vi "ZedBoardControls.vi"(4 "Register Map\nDefaults":refnum<vi>, 6 "Register Map\nRead Ref":refnum<vi>, 7 "NewRegMapReady":refnum<vi>, 8 "Last Command\nSent Ref":refnum<vi>, 9 "Stop Loop \nRef":refnum<vi>, 10 "error out":errorcluster, 11 "queue out":refnum<queue>) -> ()   [LabVIEW 2012]
panel:
  in  "Power Pulse\nReject Config":u16
  in  "Power Mon \nAcc Mode":string(combo)
  in  "Power Mon Test Mode":string(combo)
  in  "Power Mon Chan Enable":bool[](array[boolean])
  out "word9":string
  in  "Send Word A":bool
  in  "SoftDEMUX \nSelector Enable":bool
  in  "Sync Select 3B":string(combo)
  in  "Sync Select 2B":string(combo)
  in  "Sync Select 1B":string(combo)
  in  "Sync Select 0B":string(combo)
  in  "Sync Select 7":string(combo)
  in  "Sync Select 6":string(combo)
  in  "Sync Select 5":string(combo)
  in  "Sync Select 4":string(combo)
  in  "Sync Select 3A":string(combo)
  in  "Sync Select 2A":string(combo)
  in  "Sync Select 1A":string(combo)
  in  "Sync Select 0A":string(combo)
  in  "Sync Test\nMode Config":u32
  in  "Pulse Period\n(clock cycles -1)":u32
  in  "Channel DEMUX \nSelector":bool
  in  "Channel \nHold Order":bool
  in  "Channel \nTransfer Order":bool
  in  "Throttle Mode":string(combo)
  in  "Sync Test Mode Select":string(combo)
  in  "Data Input Test Mode":string(combo)
  out "Last Command Sent":string
  in  "Reset Channel Enable":bool
  in  "Send Command, manual entry":string
  in  "Send":bool
  in  "Read Register":bool
  in  "Reset Register Map to Defaults":bool
  in  "Sync Enable":bool[](array[boolean])
  in  "Channel Enable":bool[](array[boolean])
  in  "Reset Profile Accumulator":bool[](array[boolean])
  in  "Counts Per Bin":u16
  in  "User Reset":bool
  in  "Number of Bins":u16
  in  "Profiles Per Histogram":u16
  in  "Time Reset":bool
  in  "Relative Time Step":u32
  in  "Demux Channel Enable":bool[](array[boolean])
  out "word0":string
  out "word1":string
  out "word2":string
  out "word3":string
  out "word4":string
  out "word5":string
  out "word6":string
  out "word7":string
  out "word8":string
  in  "DIN Polarity":bool[](array[boolean])
  in  "DIN Demux Polarity":bool[](array[boolean])
  in  "Sync Input Polarity":bool[](array[boolean])
  in  "PIN0 Pulse Durration Ave 2^N":u16
  out "wordA":string
  in  "PIN1 Pulse Durration Ave 2^N":u16
  in  "PIN2 Pulse Durration Ave 2^N":u16
  in  "PIN3 Pulse Durration Ave 2^N":u16
  in  "PIN4 Pulse Durration Ave 2^N":u16
  in  "PIN5 Pulse Durration Ave 2^N":u16
  in  "Send Word 0":bool
  in  "Send Word 1":bool
  in  "Send Word 2":bool
  in  "Send Word 3":bool
  in  "Send Word 4":bool
  in  "Send Word 5":bool
  in  "Send Word 6":bool
  in  "Send Word 7":bool
  in  "Send Word 8":bool
  in  "Send Word 9":bool
  # "word0"
  # "word1"
  # "word2"
  # "word3"
  # "word4"
  # "valid range (2-4096)"
  # "valid range (2-4096)"
  # "valid range (1-32,768)"
  # "word5"
  # "word6"
  # "valid range (0-256)"
  # "valid range (0-64)"
  # "word7"
  # "word8"
  # "word9"
  # "valid range (0-33,554,432)"
  # "valid range (0-256)"
  # "wordA"
  # "N=valid range (0-15)"
  # "N=valid range (0-15)"
  # "N=valid range (0-15)"
  # "N=valid range (0-15)"
  # "N=valid range (0-15)"
  # "N=valid range (0-15)"
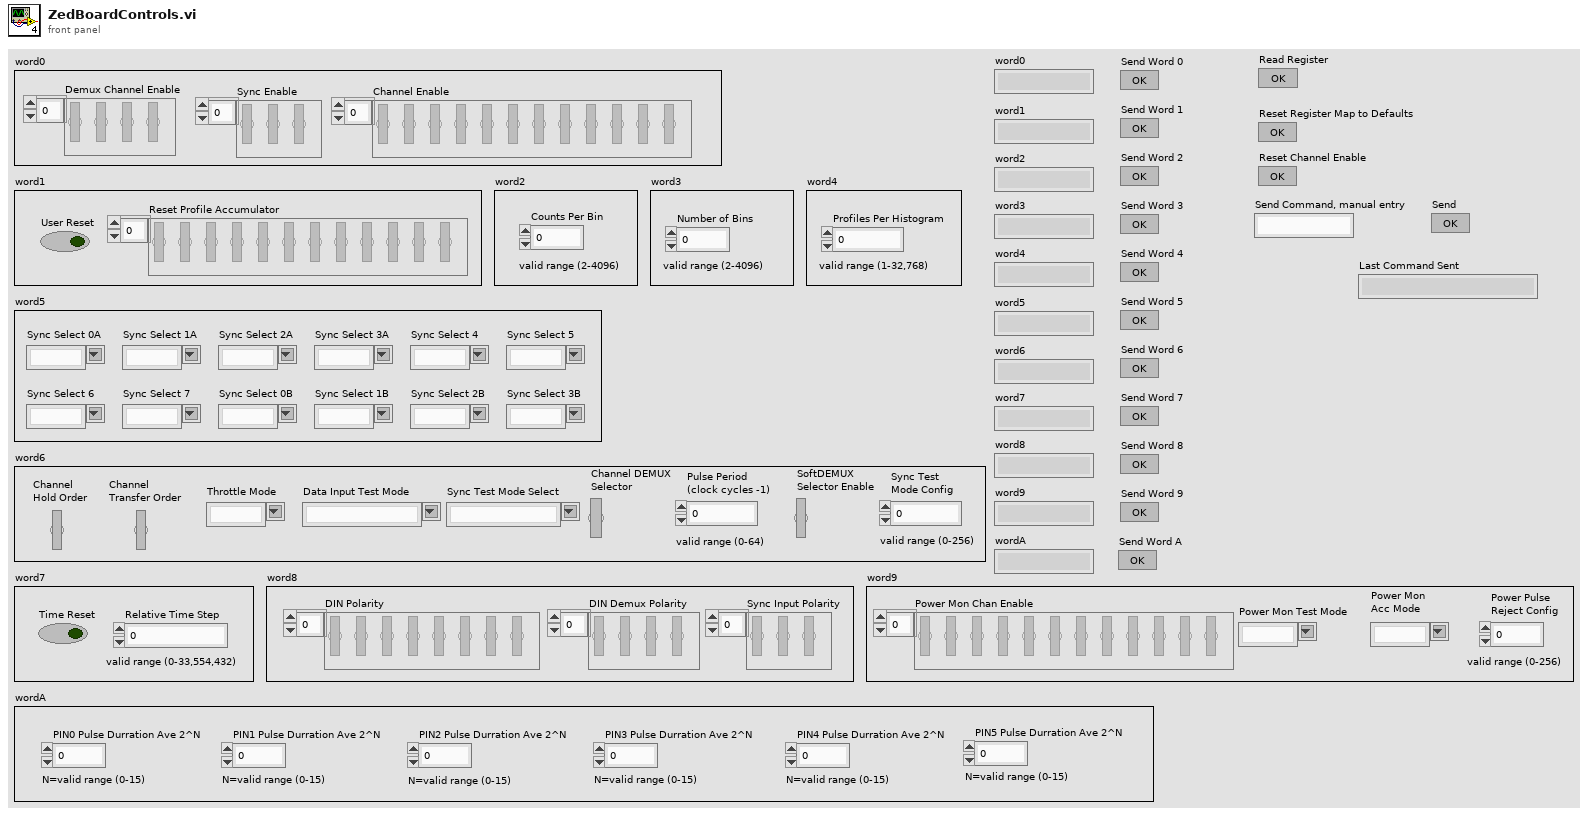
[diagram p1: front panel]
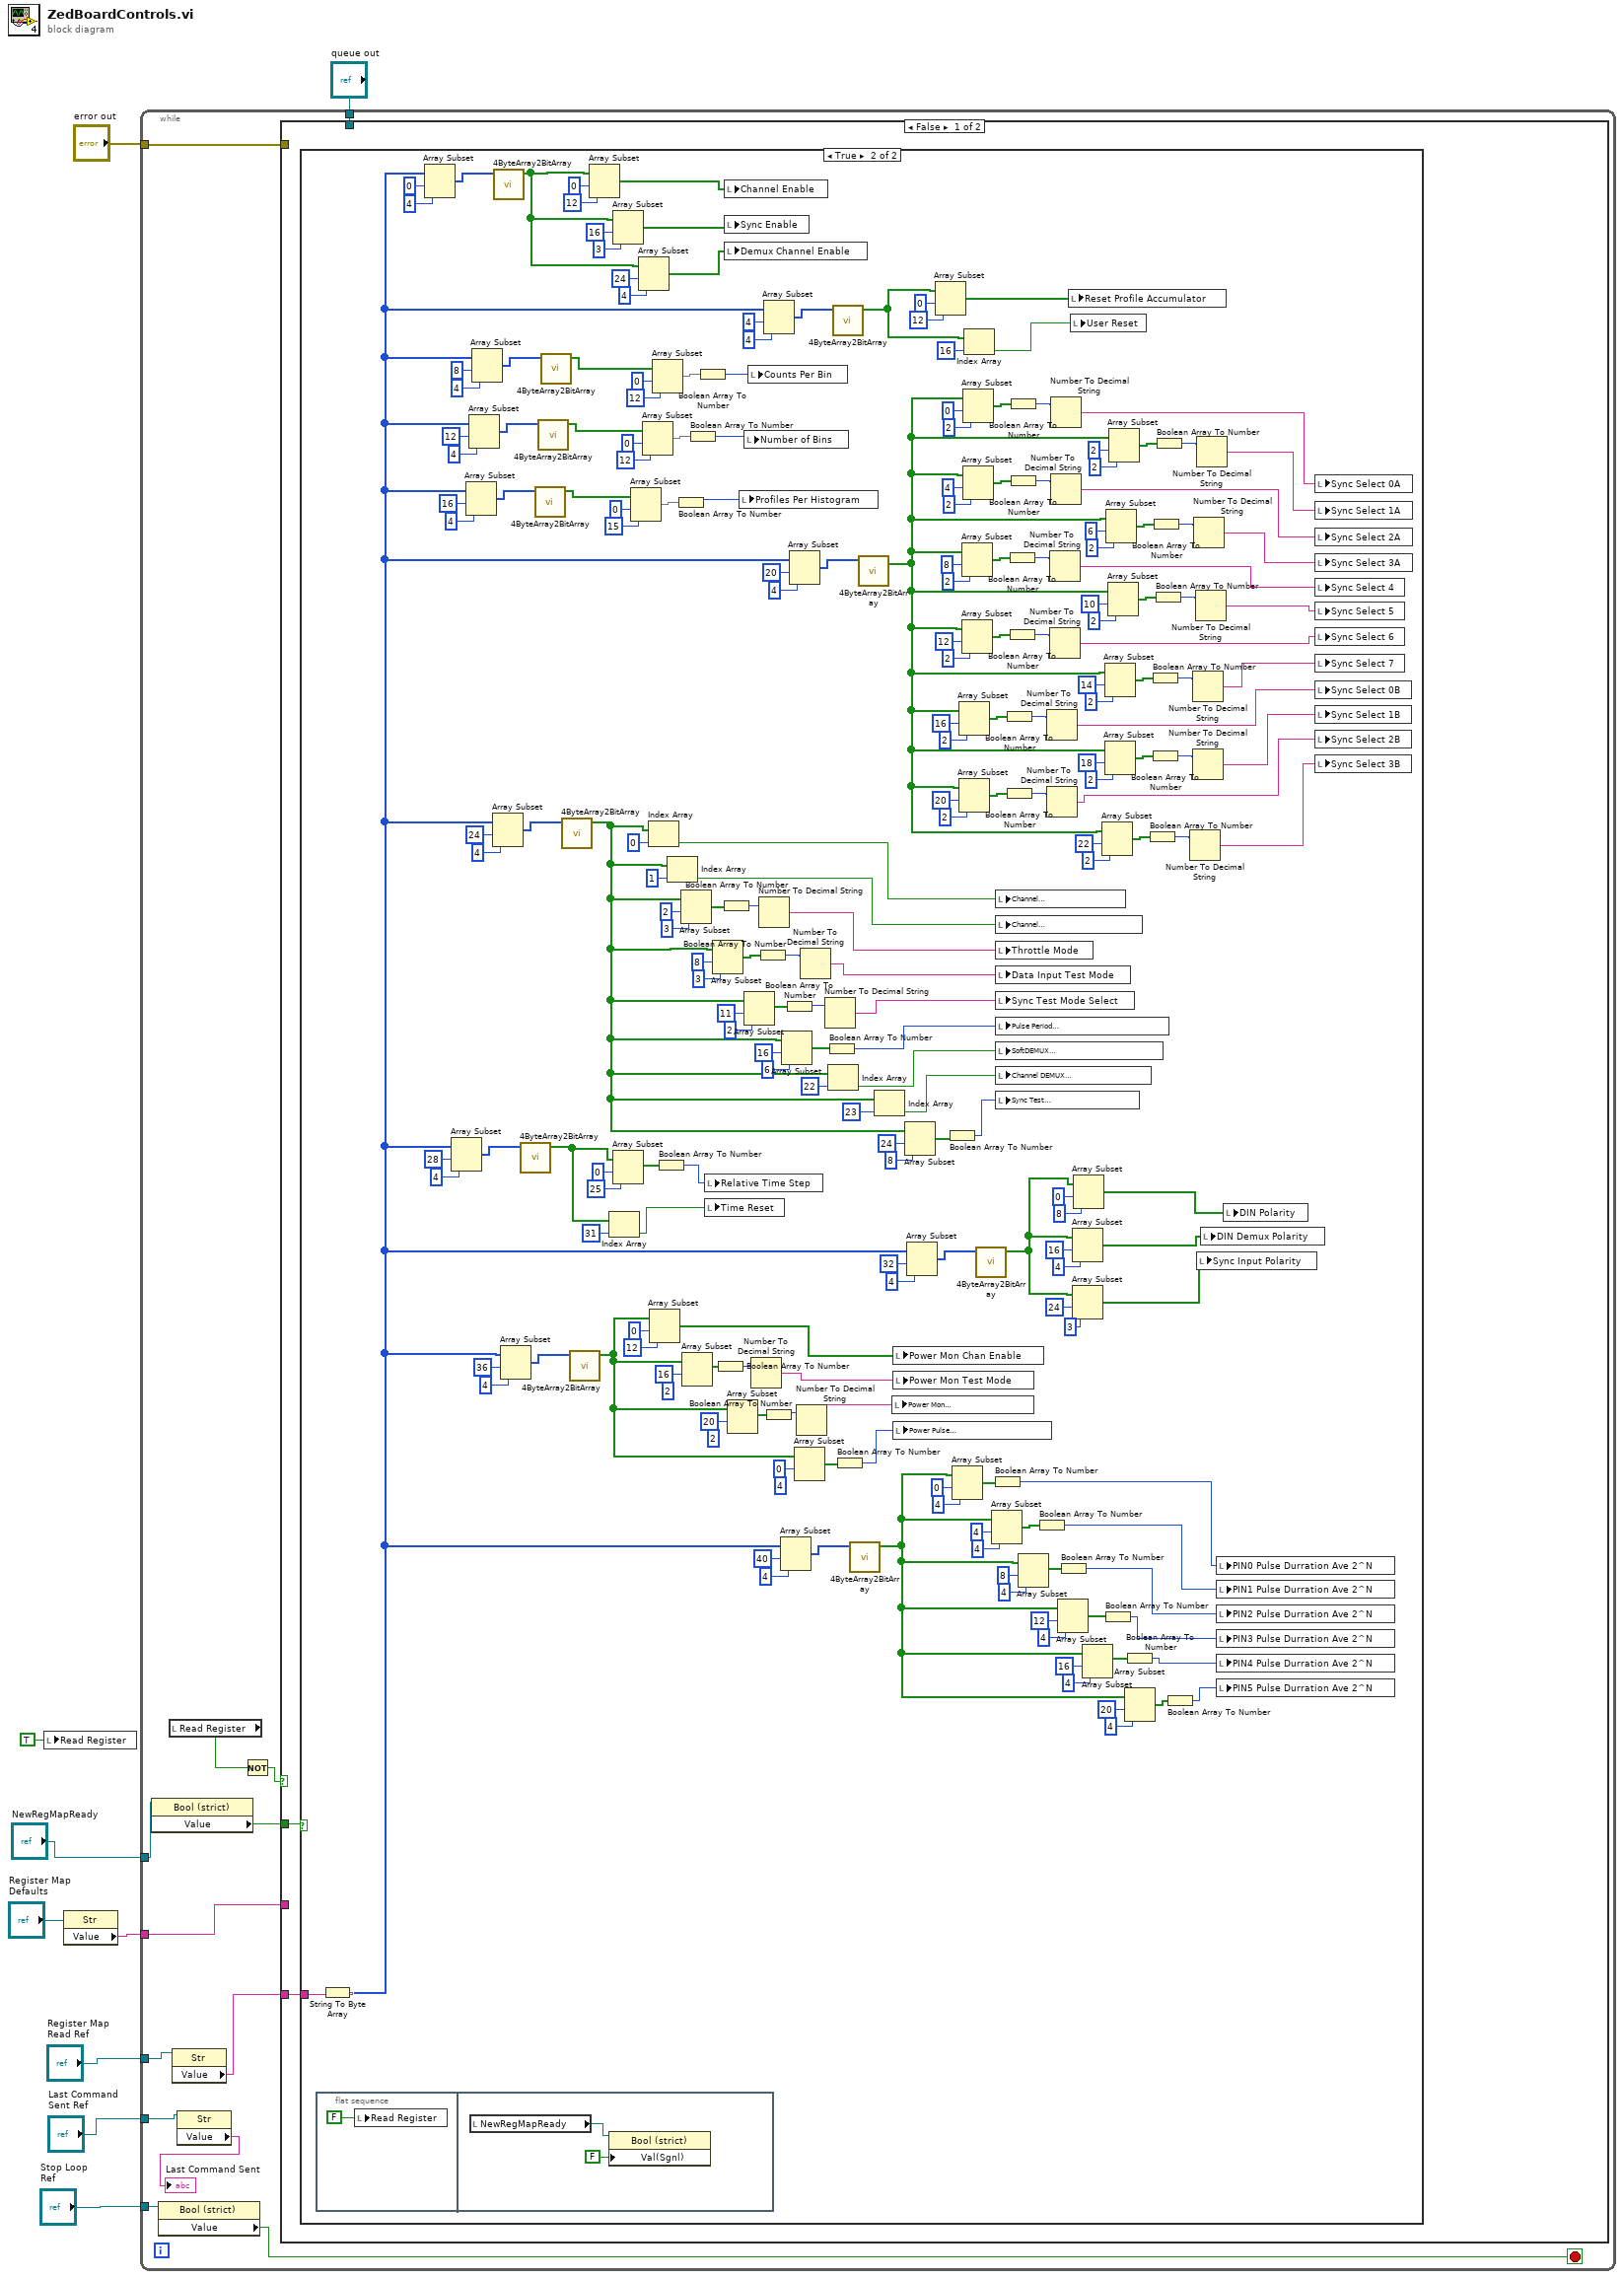
[diagram p0: block diagram]
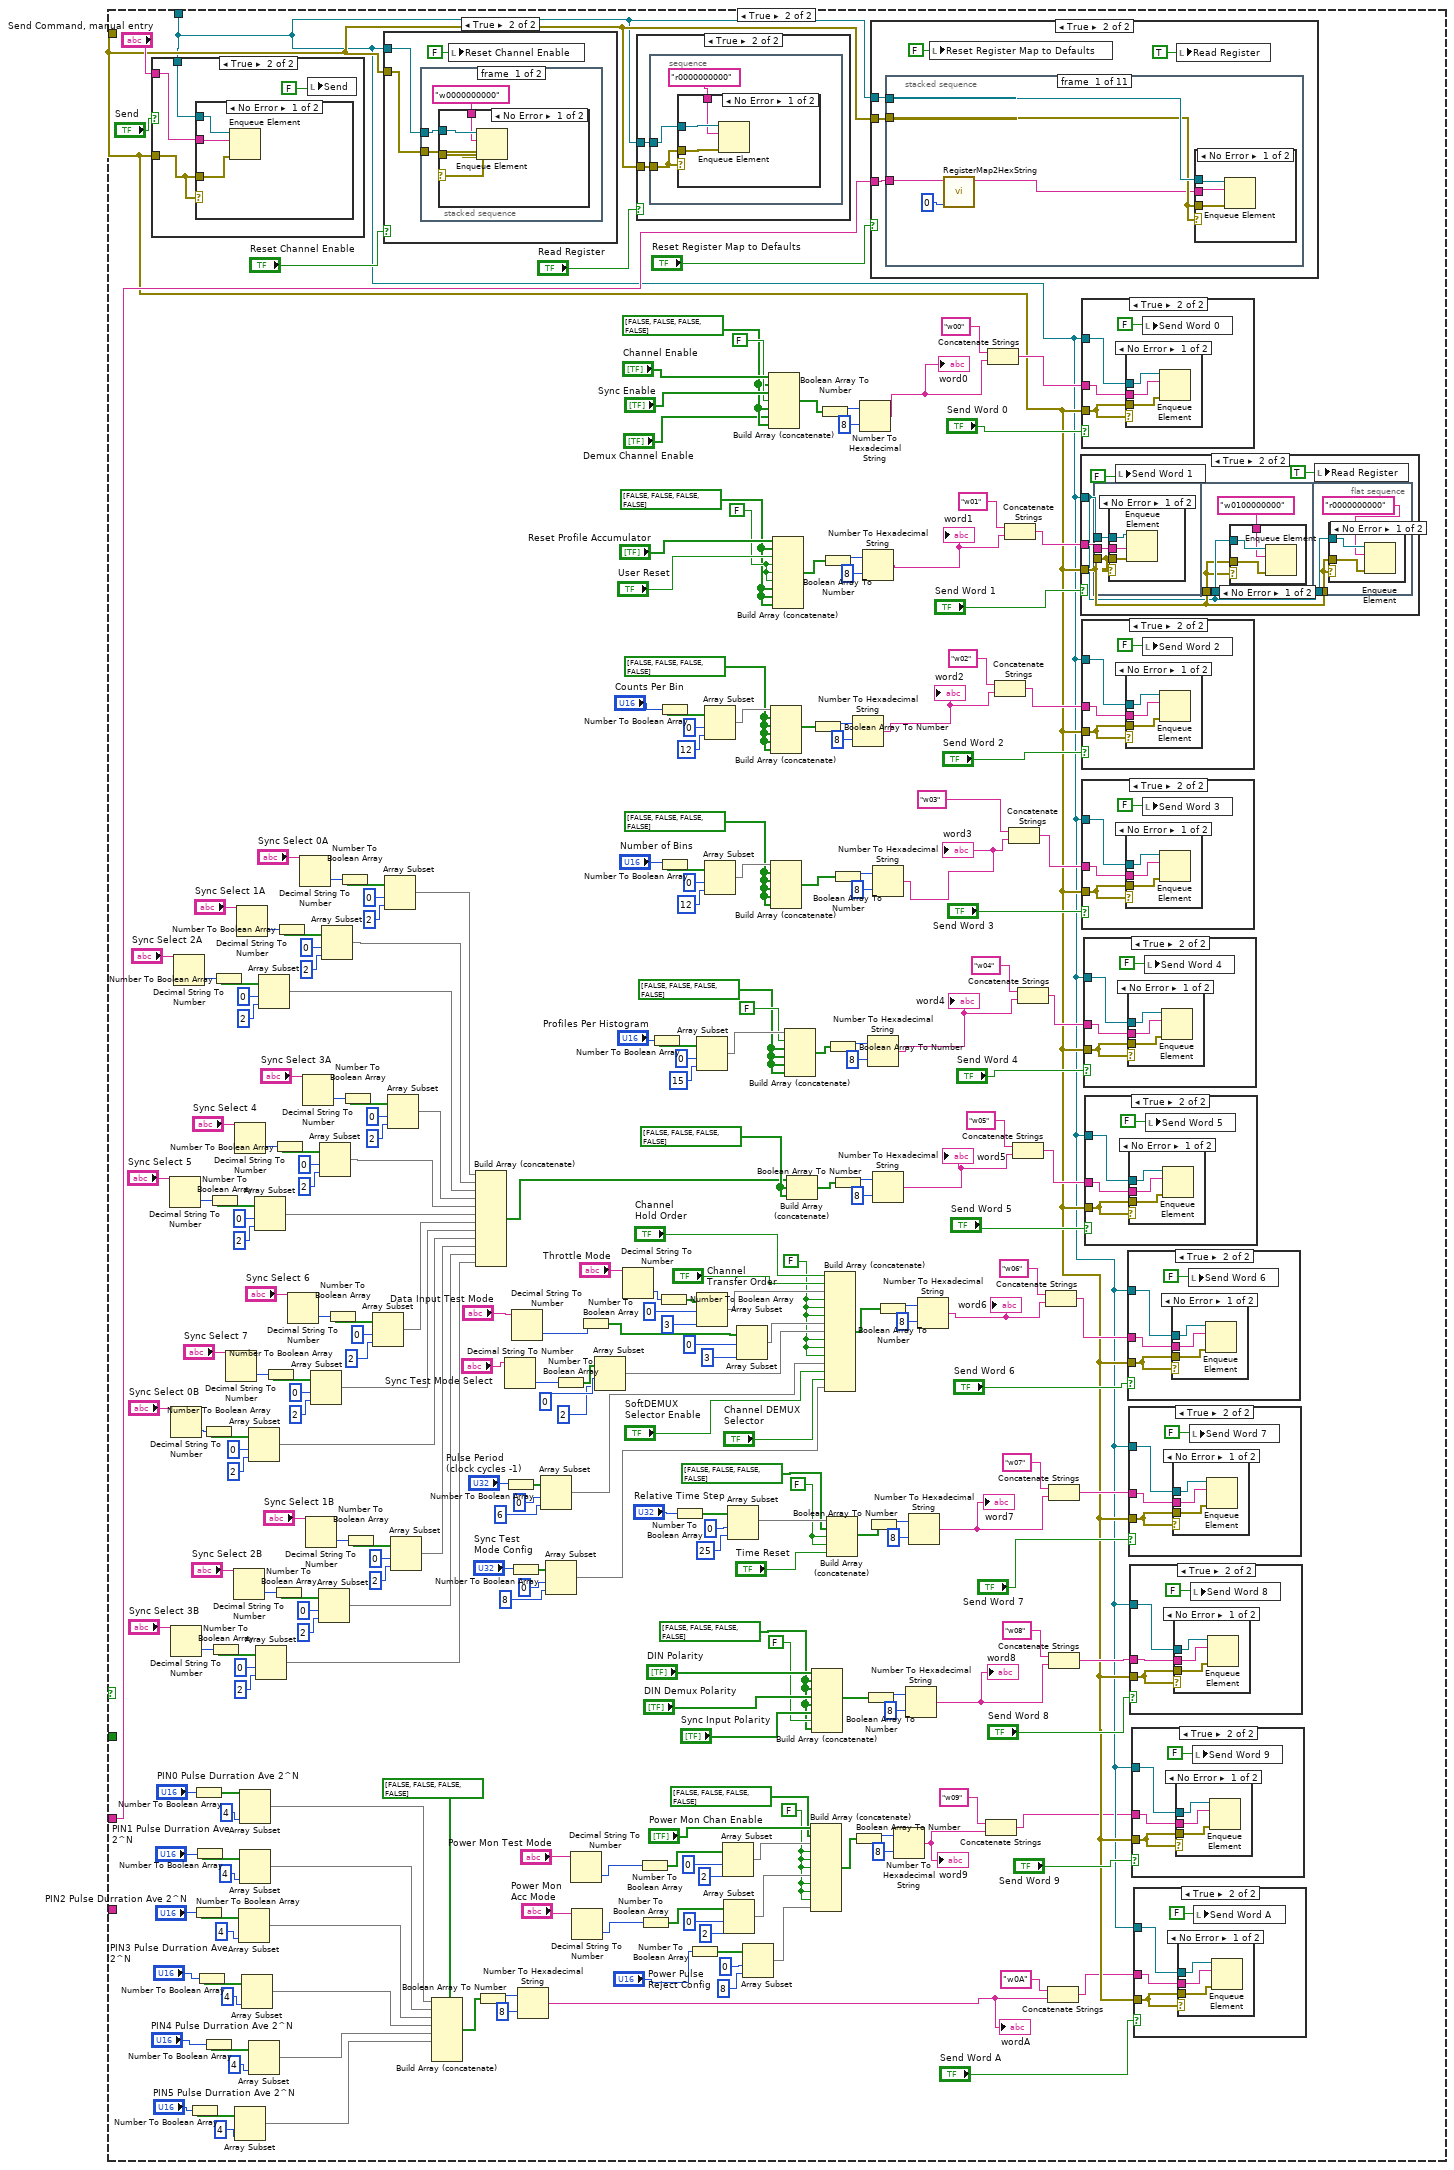
[diagram p3: hidden frame]
diagram:
  n1 = local write "Read Register"(TRUE ("Read Register")) -> ()
  n2 = property class="Str"(reference="Register Map\nDefaults") -> ("Value"=w1:string)  [unwired: 1 in, 2 out]
  n3 = while {
    tunnel: "queue out" -> [w22]
    tunnel: "error out" -> [w21]
    tunnel: "Stop Loop \nRef" -> [w20]
    tunnel: "Last Command\nSent Ref" -> [w16]
    tunnel: "Register Map\nRead Ref" -> [w17]
    tunnel: w1 -> [w13]
    tunnel: "NewRegMapReady" -> [w14]
    stop <- w19 stop-if-true
    n4 = property class="Bool (strict)"(reference=w14) -> ("Value"=w10:bool)  [unwired: 1 in, 2 out]
    n5 = property class="Bool (strict)"(reference=w20) -> ("Value"=w19:bool)  [unwired: 1 in, 2 out]
    n6 = local read "Read Register"() -> (w11:bool)
    n7 = property class="Str"(reference=w17) -> ("Value"=w15:string)  [unwired: 1 in, 2 out]
    n8 = property class="Str"(reference=w16) -> ("Value"=→"Last Command Sent":string)  [unwired: 1 in, 2 out]
    n9 = Not(x=w11) -> (.not. x?=w12:bool)
    n10 = case shown="False" w12 {
      tunnel: w22 -> [_ w270]
      tunnel: w21 -> [_ w272]
      tunnel: w15 -> [w24 _]
      tunnel: w13 -> [_ w278]
      tunnel: w10 -> [w23 _]
      frame False {
        n11 = case shown="True" w23 {
          tunnel: w24 -> [_ w240]
          frame False {
          }
          frame True {
            (unwired) 4 ("length")
            (unwired) 2 ("length")
            (unwired) 2 ("length")
            n12 = flat-sequence {
              frame #0 {
                n13 = local write "Read Register"(FALSE ("Read Register")) -> ()
              }
              frame #1 {
                n14 = local read "NewRegMapReady"() -> (w243:refnum<vi>)
                n15 = property class="Bool (strict)"(reference=w243, "Val(Sgnl)"=FALSE ("Value (Signaling)")) -> ()  [unwired: 1 in, 2 out]
              }
            }
            n16 = String To Byte Array(string=w240) -> (unsigned byte array=w40:u8[])
            n17 = Array Subset(array=w40, index=0, length=4) -> (w207:u8[])
            n18 = Array Subset(array=w40, index=28, length=4) -> (w213:u8[])
            n19 = Array Subset(array=w40, index=16, length=4) -> (w222:u8[])
            n20 = Array Subset(array=w40, index=12, length=4) -> (w225:u8[])
            n21 = Array Subset(array=w40, index=8, length=4) -> (w228:u8[])
            n22 = Array Subset(array=w40, index=24, length=4) -> (w216:u8[])
            n23 = call "4ByteArray2BitArray.vi"("array"=w207) -> ("Array"=w49:bool[])  [unwired: 10 in]
            n24 = Array Subset(array=w40, index=36, length=4) -> (w41:u8[])
            n25 = call "4ByteArray2BitArray.vi"("array"=w213) -> ("Array"=w169:bool[])  [unwired: 10 in]
            n26 = call "4ByteArray2BitArray.vi"("array"=w222) -> ("Array"=w71:bool[])  [unwired: 10 in]
            n27 = call "4ByteArray2BitArray.vi"("array"=w225) -> ("Array"=w66:bool[])  [unwired: 10 in]
            n28 = call "4ByteArray2BitArray.vi"("array"=w228) -> ("Array"=w61:bool[])  [unwired: 10 in]
            n29 = call "4ByteArray2BitArray.vi"("array"=w216) -> ("Array"=w46:bool[])  [unwired: 10 in]
            n30 = call "4ByteArray2BitArray.vi"("array"=w41) -> ("Array"=w26:bool[])  [unwired: 10 in]
            n31 = Array Subset(array=w49, index=0, length=12) -> (w237:bool[])
            n32 = Index Array(array=w169, index=31) -> (element=w167:bool)
            n33 = Array Subset(array=w49, index=16, length=3) -> (w48:bool[])
            n34 = Array Subset(array=w169, index=0, length=25) -> (w165:bool[])
            n35 = Array Subset(array=w71, index=0, length=15) -> (w72:bool[])
            n36 = Array Subset(array=w49, index=24, length=4) -> (w47:bool[])
            n37 = Array Subset(array=w66, index=0, length=12) -> (w67:bool[])
            n38 = Index Array(array=w46, index=0) -> (element=w147:bool)
            n39 = Array Subset(array=w26, index=0, length=12) -> (w37:bool[])
            n40 = Array Subset(array=w61, index=0, length=12) -> (w62:bool[])
            n41 = Boolean Array To Number(Boolean array=w165) -> (number=w166:u32)
            n42 = Index Array(array=w46, index=1) -> (element=w146:bool)
            n43 = Boolean Array To Number(Boolean array=w72) -> (number=w70:u32)
            n44 = Array Subset(array=w46, index=2, length=3) -> (w153:bool[])
            n45 = Array Subset(array=w26, index=16) -> (w35:bool[])  [unwired: 1 in]
            n46 = Boolean Array To Number(Boolean array=w67) -> (number=w65:u32)
            n47 = Boolean Array To Number(Boolean array=w62) -> (number=w60:u32)
            n48 = local write "Relative Time Step"(w166) -> ()
            n49 = local write "Time Reset"(w167) -> ()
            n50 = Array Subset(array=w46, index=8, length=3) -> (w154:bool[])
            n51 = Boolean Array To Number(Boolean array=w35) -> (number=w34:u32)
            n52 = Boolean Array To Number(Boolean array=w153) -> (number=w145:u32)
            n53 = local write "Channel Enable"(w237) -> ()
            n54 = local write "Sync Enable"(w48) -> ()
            n55 = local write "Demux Channel Enable"(w47) -> ()
            n56 = Array Subset(array=w26, index=20) -> (w31:bool[])  [unwired: 1 in]
            n57 = local write "Profiles Per Histogram"(w70) -> ()
            n58 = local write "Number of Bins"(w65) -> ()
            n59 = Array Subset(array=w46, index=11, length=2) -> (w152:bool[])
            n60 = local write "Counts Per Bin"(w60) -> ()
            n61 = Number To Decimal String(number=w34) -> (decimal integer string=w33:string)  [unwired: 1 in]
            n62 = Boolean Array To Number(Boolean array=w154) -> (number=w143:u32)
            n63 = Number To Decimal String(number=w145) -> (decimal integer string=w144:string)  [unwired: 1 in]
            n64 = Array Subset(array=w40, index=4, length=4) -> (w231:u8[])
            n65 = Boolean Array To Number(Boolean array=w31) -> (number=w30:u32)
            n66 = Array Subset(array=w40, index=40, length=4) -> (w234:u8[])
            n67 = Array Subset(array=w46, index=16, length=6) -> (w151:bool[])
            n68 = Boolean Array To Number(Boolean array=w152) -> (number=w141:u32)
            n69 = Array Subset(array=w40, index=20, length=4) -> (w219:u8[])
            n70 = Array Subset(array=w26, index=0) -> (w27:bool[])  [unwired: 1 in]
            n71 = Number To Decimal String(number=w30) -> (decimal integer string=w29:string)  [unwired: 1 in]
            n72 = Number To Decimal String(number=w143) -> (decimal integer string=w142:string)  [unwired: 1 in]
            n73 = Number To Decimal String(number=w141) -> (decimal integer string=w140:string)  [unwired: 1 in]
            n74 = Boolean Array To Number(Boolean array=w151) -> (number=w137:u32)
            n75 = Index Array(array=w46, index=22) -> (element=w44:bool)
            n76 = call "4ByteArray2BitArray.vi"("array"=w231) -> ("Array"=w56:bool[])  [unwired: 10 in]
            n77 = Boolean Array To Number(Boolean array=w27) -> (number=w25:u32)
            n78 = call "4ByteArray2BitArray.vi"("array"=w234) -> ("Array"=w194:bool[])  [unwired: 10 in]
            n79 = call "4ByteArray2BitArray.vi"("array"=w219) -> ("Array"=w87:bool[])  [unwired: 10 in]
            n80 = Index Array(array=w46, index=23) -> (element=w138:bool)
            n81 = local write "Power Mon \nAcc Mode"(w29) -> ()
            n82 = local write "Power Mon Chan Enable"(w37) -> ()
            n83 = local write "Power Mon Test Mode"(w33) -> ()
            n84 = local write "Power Pulse\nReject Config"(w25) -> ()
            n85 = Array Subset(array=w46, index=24, length=8) -> (w150:bool[])
            n86 = Array Subset(array=w40, index=32, length=4) -> (w210:u8[])
            n87 = Array Subset(array=w56, index=0, length=12) -> (w55:bool[])
            n88 = Boolean Array To Number(Boolean array=w150) -> (number=w136:u32)
            n89 = Array Subset(array=w194, index=0, length=4) -> (w191:bool[])
            n90 = Array Subset(array=w87, index=16, length=2) -> (w101:bool[])
            n91 = Array Subset(array=w87, index=20, length=2) -> (w93:bool[])
            n92 = Array Subset(array=w87, index=8, length=2) -> (w117:bool[])
            n93 = Array Subset(array=w87, index=12, length=2) -> (w109:bool[])
            n94 = Array Subset(array=w87, index=0, length=2) -> (w133:bool[])
            n95 = Array Subset(array=w87, index=4, length=2) -> (w125:bool[])
            n96 = Index Array(array=w56, index=16) -> (element=w54:bool)
            n97 = call "4ByteArray2BitArray.vi"("array"=w210) -> ("Array"=w175:bool[])  [unwired: 10 in]
            n98 = Array Subset(array=w194, index=4, length=4) -> (w193:bool[])
            n99 = Boolean Array To Number(Boolean array=w191) -> (number=w190:u32)
            n100 = local write "Channel \nHold Order"(w147) -> ()
            n101 = local write "Channel \nTransfer Order"(w146) -> ()
            n102 = local write "Throttle Mode"(w144) -> ()
            n103 = local write "Data Input Test Mode"(w142) -> ()
            n104 = local write "Sync Test Mode Select"(w140) -> ()
            n105 = local write "Pulse Period\n(clock cycles -1)"(w137) -> ()
            n106 = local write "SoftDEMUX \nSelector Enable"(w44) -> ()
            n107 = local write "Channel DEMUX \nSelector"(w138) -> ()
            n108 = local write "Sync Test\nMode Config"(w136) -> ()
            n109 = Boolean Array To Number(Boolean array=w101) -> (number=w100:u32)
            n110 = Boolean Array To Number(Boolean array=w93) -> (number=w92:u32)
            n111 = Boolean Array To Number(Boolean array=w117) -> (number=w116:u32)
            n112 = Boolean Array To Number(Boolean array=w109) -> (number=w108:u32)
            n113 = Boolean Array To Number(Boolean array=w133) -> (number=w132:u32)
            n114 = Boolean Array To Number(Boolean array=w125) -> (number=w124:u32)
            n115 = Array Subset(array=w194, index=8, length=4) -> (w188:bool[])
            n116 = Boolean Array To Number(Boolean array=w193) -> (number=w192:u32)
            n117 = Number To Decimal String(number=w100) -> (decimal integer string=w78:string)  [unwired: 1 in]
            n118 = Number To Decimal String(number=w92) -> (decimal integer string=w76:string)  [unwired: 1 in]
            n119 = Number To Decimal String(number=w116) -> (decimal integer string=w82:string)  [unwired: 1 in]
            n120 = Number To Decimal String(number=w108) -> (decimal integer string=w80:string)  [unwired: 1 in]
            n121 = Number To Decimal String(number=w132) -> (decimal integer string=w86:string)  [unwired: 1 in]
            n122 = Number To Decimal String(number=w124) -> (decimal integer string=w84:string)  [unwired: 1 in]
            n123 = Array Subset(array=w194, index=12, length=4) -> (w187:bool[])
            n124 = Boolean Array To Number(Boolean array=w188) -> (number=w189:u32)
            n125 = local write "Reset Profile Accumulator"(w55) -> ()
            n126 = local write "User Reset"(w54) -> ()
            n127 = Array Subset(array=w175, index=16, length=4) -> (w172:bool[])
            n128 = Array Subset(array=w175, index=24, length=3) -> (w173:bool[])
            n129 = Array Subset(array=w175, index=0, length=8) -> (w174:bool[])
            n130 = Array Subset(array=w194, index=16, length=4) -> (w186:bool[])
            n131 = Array Subset(array=w87, index=22, length=2) -> (w89:bool[])
            n132 = Boolean Array To Number(Boolean array=w187) -> (number=w182:u32)
            n133 = Array Subset(array=w87, index=14, length=2) -> (w105:bool[])
            n134 = Array Subset(array=w87, index=18, length=2) -> (w97:bool[])
            n135 = Array Subset(array=w87, index=6, length=2) -> (w121:bool[])
            n136 = Array Subset(array=w87, index=10, length=2) -> (w113:bool[])
            n137 = Array Subset(array=w87, index=2, length=2) -> (w129:bool[])
            n138 = Boolean Array To Number(Boolean array=w186) -> (number=w183:u32)
            n139 = Array Subset(array=w194, index=20, length=4) -> (w185:bool[])
            n140 = Boolean Array To Number(Boolean array=w89) -> (number=w88:u32)
            n141 = Boolean Array To Number(Boolean array=w105) -> (number=w104:u32)
            n142 = Boolean Array To Number(Boolean array=w97) -> (number=w96:u32)
            n143 = Boolean Array To Number(Boolean array=w121) -> (number=w120:u32)
            n144 = Boolean Array To Number(Boolean array=w113) -> (number=w112:u32)
            n145 = Boolean Array To Number(Boolean array=w129) -> (number=w128:u32)
            n146 = Boolean Array To Number(Boolean array=w185) -> (number=w184:u32)
            n147 = Number To Decimal String(number=w88) -> (decimal integer string=w75:string)  [unwired: 1 in]
            n148 = Number To Decimal String(number=w104) -> (decimal integer string=w79:string)  [unwired: 1 in]
            n149 = Number To Decimal String(number=w96) -> (decimal integer string=w77:string)  [unwired: 1 in]
            n150 = Number To Decimal String(number=w120) -> (decimal integer string=w83:string)  [unwired: 1 in]
            n151 = Number To Decimal String(number=w112) -> (decimal integer string=w81:string)  [unwired: 1 in]
            n152 = Number To Decimal String(number=w128) -> (decimal integer string=w85:string)  [unwired: 1 in]
            n153 = local write "Sync Input Polarity"(w173) -> ()
            n154 = local write "DIN Demux Polarity"(w172) -> ()
            n155 = local write "PIN0 Pulse Durration Ave 2^N"(w190) -> ()
            n156 = local write "PIN1 Pulse Durration Ave 2^N"(w192) -> ()
            n157 = local write "PIN2 Pulse Durration Ave 2^N"(w189) -> ()
            n158 = local write "PIN3 Pulse Durration Ave 2^N"(w182) -> ()
            n159 = local write "PIN4 Pulse Durration Ave 2^N"(w183) -> ()
            n160 = local write "PIN5 Pulse Durration Ave 2^N"(w184) -> ()
            n161 = local write "DIN Polarity"(w174) -> ()
            n162 = local write "Sync Select 0A"(w86) -> ()
            n163 = local write "Sync Select 1A"(w85) -> ()
            n164 = local write "Sync Select 2A"(w84) -> ()
            n165 = local write "Sync Select 3A"(w83) -> ()
            n166 = local write "Sync Select 4"(w82) -> ()
            n167 = local write "Sync Select 5"(w81) -> ()
            n168 = local write "Sync Select 6"(w80) -> ()
            n169 = local write "Sync Select 7"(w79) -> ()
            n170 = local write "Sync Select 0B"(w78) -> ()
            n171 = local write "Sync Select 1B"(w77) -> ()
            n172 = local write "Sync Select 2B"(w76) -> ()
            n173 = local write "Sync Select 3B"(w75) -> ()
          }
        }
      }
      frame True {
        w249 = FALSE ("Read Register")
        w450 = bool[] [FALSE, FALSE, FALSE, FALSE] ("appended array")
        w474 = bool[] [FALSE, FALSE, FALSE, FALSE] ("appended array")
        w480 = FALSE ("Read Register")
        w399 = FALSE ("Read Register")
        w485 = bool[] [FALSE, FALSE, FALSE, FALSE] ("appended array")
        w320 = bool[] [FALSE, FALSE, FALSE, FALSE] ("appended array")
        w483 = bool[] [FALSE, FALSE, FALSE, FALSE] ("appended array")
        w484 = bool[] [FALSE, FALSE, FALSE, FALSE] ("appended array")
        w498 = FALSE ("Read Register")
        w497 = bool[] [FALSE, FALSE, FALSE, FALSE] ("appended array")
        w502 = bool[] [FALSE, FALSE, FALSE, FALSE] ("appended array")
        n174 = case shown="True" "Send" {
          tunnel: "Send Command, manual entry" -> [_ w732]
          tunnel: w270 -> [_ w731]
          tunnel: w272 -> [_ w729]
          frame False {
          }
          frame True {
            n175 = case shown="No Error" w729 {
              tunnel: w732 -> [w735 _]
              tunnel: w729 -> [w734 _]
              tunnel: w731 -> [w733 _]
              frame No Error {
                n176 = Enqueue Element(queue=w733, element=w735, error in (no error)=w734) -> ()  [unwired: 1 in, 3 out]
              }
              frame Error {
              }
            }
            n177 = local write "Send"(FALSE ("Send")) -> ()
          }
        }
        n178 = Decimal String To Number(string="Sync Select 5") -> (number=w364:i32)  [unwired: 2 in, 1 out]
        n179 = Decimal String To Number(string="Sync Select 0B") -> (number=w349:i32)  [unwired: 2 in, 1 out]
        n180 = Decimal String To Number(string="Sync Select 3B") -> (number=w334:i32)  [unwired: 2 in, 1 out]
        n181 = Decimal String To Number(string="Sync Select 2A") -> (number=w379:i32)  [unwired: 2 in, 1 out]
        n182 = Number To Boolean Array(number="PIN5 Pulse Durration Ave 2^N") -> (Boolean array=w466:bool[])
        n183 = Number To Boolean Array(number="PIN0 Pulse Durration Ave 2^N") -> (Boolean array=w472:bool[])
        n184 = Number To Boolean Array(number="PIN2 Pulse Durration Ave 2^N") -> (Boolean array=w462:bool[])
        n185 = Number To Boolean Array(number="PIN1 Pulse Durration Ave 2^N") -> (Boolean array=w470:bool[])
        n186 = Number To Boolean Array(number="PIN3 Pulse Durration Ave 2^N") -> (Boolean array=w464:bool[])
        n187 = Number To Boolean Array(number=w349) -> (Boolean array=w351:bool[])
        n188 = Number To Boolean Array(number="PIN4 Pulse Durration Ave 2^N") -> (Boolean array=w468:bool[])
        n189 = Number To Boolean Array(number=w364) -> (Boolean array=w366:bool[])
        n190 = Number To Boolean Array(number=w334) -> (Boolean array=w336:bool[])
        n191 = Number To Boolean Array(number=w379) -> (Boolean array=w381:bool[])
        n192 = Decimal String To Number(string="Sync Select 7") -> (number=w354:i32)  [unwired: 2 in, 1 out]
        n193 = Decimal String To Number(string="Sync Select 2B") -> (number=w339:i32)  [unwired: 2 in, 1 out]
        n194 = Decimal String To Number(string="Sync Select 4") -> (number=w369:i32)  [unwired: 2 in, 1 out]
        n195 = Array Subset(array=w466, length=4) -> (w451:bool[])  [unwired: 1 in]
        n196 = Decimal String To Number(string="Sync Select 1A") -> (number=w384:i32)  [unwired: 2 in, 1 out]
        n197 = Array Subset(array=w462, length=4) -> (w454:bool[])  [unwired: 1 in]
        n198 = Array Subset(array=w472, length=4) -> (w456:bool[])  [unwired: 1 in]
        n199 = Array Subset(array=w470, length=4) -> (w455:bool[])  [unwired: 1 in]
        n200 = Array Subset(array=w464, length=4) -> (w453:bool[])  [unwired: 1 in]
        n201 = Array Subset(array=w351, index=0, length=2) -> (w324:bool[])
        n202 = Array Subset(array=w468, length=4) -> (w452:bool[])  [unwired: 1 in]
        n203 = Array Subset(array=w366, index=0, length=2) -> (w328:bool[])
        n204 = Array Subset(array=w336, index=0, length=2) -> (w327:bool[])
        n205 = Array Subset(array=w381, index=0, length=2) -> (w331:bool[])
        n206 = Number To Boolean Array(number=w354) -> (Boolean array=w356:bool[])
        n207 = Number To Boolean Array(number=w339) -> (Boolean array=w341:bool[])
        n208 = Number To Boolean Array(number=w369) -> (Boolean array=w371:bool[])
        n209 = Number To Boolean Array(number=w384) -> (Boolean array=w386:bool[])
        n210 = Decimal String To Number(string="Sync Select 6") -> (number=w359:i32)  [unwired: 2 in, 1 out]
        n211 = Decimal String To Number(string="Sync Select 0A") -> (number=w389:i32)  [unwired: 2 in, 1 out]
        n212 = Decimal String To Number(string="Sync Select 3A") -> (number=w374:i32)  [unwired: 2 in, 1 out]
        n213 = Decimal String To Number(string="Sync Select 1B") -> (number=w344:i32)  [unwired: 2 in, 1 out]
        n214 = Array Subset(array=w356, index=0, length=2) -> (w323:bool[])
        n215 = Array Subset(array=w341, index=0, length=2) -> (w326:bool[])
        n216 = Array Subset(array=w371, index=0, length=2) -> (w329:bool[])
        n217 = Array Subset(array=w386, index=0, length=2) -> (w332:bool[])
        n218 = Number To Boolean Array(number=w359) -> (Boolean array=w361:bool[])
        n219 = Number To Boolean Array(number=w389) -> (Boolean array=w391:bool[])
        n220 = Number To Boolean Array(number=w374) -> (Boolean array=w376:bool[])
        n221 = Number To Boolean Array(number=w344) -> (Boolean array=w346:bool[])
        n222 = Array Subset(array=w361, index=0, length=2) -> (w322:bool[])
        n223 = case shown="True" "Reset Channel Enable" {
          tunnel: w272 -> [_ w714]
          tunnel: w270 -> [_ w715]
          frame False {
          }
          frame True {
            n224 = stacked-sequence {
              tunnel: w714 -> [w719 w724]
              tunnel: w715 -> [w717 w723]
              frame #0 {
                n225 = case shown="No Error" w719 {
                  tunnel: w719 -> [w722 _]
                  tunnel: w717 -> [w721 _]
                  tunnel: "w0000000000" ("F-format string") -> [w720 _]
                  frame No Error {
                    n226 = Enqueue Element(queue=w721, element=w720, error in (no error)=w722) -> ()  [unwired: 1 in, 3 out]
                  }
                  frame Error {
                  }
                }
              }
              frame #1 {
                n227 = case shown="No Error" w724 {
                  tunnel: "w0000010fff" ("F-format string") -> [w728 _]
                  tunnel: w723 -> [w727 _]
                  tunnel: w724 -> [w726 _]
                  frame No Error {
                    n228 = Enqueue Element(queue=w727, element=w728, error in (no error)=w726) -> ()  [unwired: 1 in, 3 out]
                  }
                  frame Error {
                  }
                }
              }
            }
            n229 = local write "Reset Channel Enable"(FALSE ("Reset")) -> ()
          }
        }
        n230 = Array Subset(array=w391, index=0, length=2) -> (w333:bool[])
        n231 = Array Subset(array=w376, index=0, length=2) -> (w330:bool[])
        n232 = Array Subset(array=w346, index=0, length=2) -> (w325:bool[])
        n233 = Build Array (concatenate)(w456, w455, w454, w453, w452, w451, w450, w450) -> (w280:bool[])
        n234 = Build Array (concatenate)(w333, w332, w331, w330, w329, w328, w322, w323, w324, w325, w326, w327) -> (w421:bool[])
        n235 = Boolean Array To Number(Boolean array=w280) -> (number=w298:u32)
        n236 = Decimal String To Number(string="Sync Test Mode Select") -> (number=w415:i32)  [unwired: 2 in, 1 out]
        n237 = Number To Boolean Array(number="Pulse Period\n(clock cycles -1)") -> (Boolean array=w408:bool[])
        n238 = Number To Boolean Array(number="Sync Test\nMode Config") -> (Boolean array=w398:bool[])
        n239 = Decimal String To Number(string="Data Input Test Mode") -> (number=w416:i32)  [unwired: 2 in, 1 out]
        n240 = Number To Hexadecimal String(1:i16 8 ("width (-)"), 2:w298) -> (0:w279:string)
        "wordA" <- w279
        n241 = Array Subset(array=w408, index=0, length=6) -> (w276:bool[])
        n242 = Array Subset(array=w398, index=0, length=8) -> (w277:bool[])
        n243 = Number To Boolean Array(number=w415) -> (Boolean array=w409:bool[])
        n244 = Decimal String To Number(string="Power Mon Test Mode") -> (number=w260:i32)  [unwired: 2 in, 1 out]
        n245 = Decimal String To Number(string="Power Mon \nAcc Mode") -> (number=w255:i32)  [unwired: 2 in, 1 out]
        n246 = Number To Boolean Array(number=w416) -> (Boolean array=w410:bool[])
        n247 = Array Subset(array=w409, index=0, length=2) -> (w400:bool[])
        n248 = Decimal String To Number(string="Throttle Mode") -> (number=w419:i32)  [unwired: 2 in, 1 out]
        n249 = case shown="True" "Read Register" {
          tunnel: w270 -> [_ w706]
          tunnel: w272 -> [_ w707]
          frame False {
          }
          frame True {
            n250 = stacked-sequence {
              tunnel: w707 -> [w709]
              tunnel: w706 -> [w708]
              frame #0 {
                n251 = case shown="No Error" w709 {
                  tunnel: w708 -> [w713 _]
                  tunnel: w709 -> [w712 _]
                  tunnel: "r0000000000" ("F-format string") -> [w711 _]
                  frame No Error {
                    n252 = Enqueue Element(queue=w713, element=w711, error in (no error)=w712) -> ()  [unwired: 1 in, 3 out]
                  }
                  frame Error {
                  }
                }
              }
            }
          }
        }
        n253 = Number To Boolean Array(number=w260) -> (Boolean array=w259:bool[])
        n254 = Number To Boolean Array(number=w255) -> (Boolean array=w254:bool[])
        n255 = Number To Boolean Array(number="Profiles Per Histogram") -> (Boolean array=w488:bool[])
        n256 = Number To Boolean Array(number=w419) -> (Boolean array=w511:bool[])
        n257 = Number To Boolean Array(number="Counts Per Bin") -> (Boolean array=w514:bool[])
        n258 = Number To Boolean Array(number="Number of Bins") -> (Boolean array=w493:bool[])
        n259 = Number To Boolean Array(number="Relative Time Step") -> (Boolean array=w508:bool[])
        n260 = Number To Boolean Array(number="Power Pulse\nReject Config") -> (Boolean array=w247:bool[])
        n261 = Array Subset(array=w488, index=0, length=15) -> (w487:bool[])
        n262 = Array Subset(array=w511, index=0, length=3) -> (w404:bool[])
        n263 = Array Subset(array=w514, index=0, length=12) -> (w496:bool[])
        n264 = Array Subset(array=w493, index=0, length=12) -> (w492:bool[])
        n265 = Array Subset(array=w259, index=0, length=2) -> (w256:bool[])
        n266 = Array Subset(array=w254, index=0, length=2) -> (w250:bool[])
        n267 = Array Subset(array=w508, index=0, length=25) -> (w482:bool[])
        n268 = Array Subset(array=w410, index=0, length=3) -> (w401:bool[])
        n269 = Array Subset(array=w247, index=0, length=8) -> (w244:bool[])
        n270 = Build Array (concatenate)("Channel Enable", w502, "Sync Enable", FALSE ("Read Register"), w502, "Demux Channel Enable", w502) -> (w296:bool[])
        n271 = Build Array (concatenate)(w496, w484, w484, w484, w484, w484) -> (w292:bool[])
        n272 = Build Array (concatenate)(w492, w483, w483, w483, w483, w483) -> (w315:bool[])
        n273 = Build Array (concatenate)("Reset Profile Accumulator", w497, "User Reset", w498, w498, w498, w497, w497, w497) -> (w294:bool[])
        n274 = Build Array (concatenate)(w487, FALSE ("Read Register"), w320, w320, w320, w320) -> (w290:bool[])
        n275 = Build Array (concatenate)(w421, w485, w485) -> (w288:bool[])
        n276 = Build Array (concatenate)("Power Mon Chan Enable", bool[] [FALSE, FALSE, FALSE, FALSE] ("appended array"), w256, w249, w249, w249, w250, w249, w249, w249, w244) -> (w264:bool[])
        n277 = Build Array (concatenate)("DIN Polarity", w474, w474, "DIN Demux Polarity", w474, "Sync Input Polarity", FALSE ("Read Register"), w474) -> (w282:bool[])
        n278 = Boolean Array To Number(Boolean array=w292) -> (number=w310:u32)
        n279 = Boolean Array To Number(Boolean array=w296) -> (number=w314:u32)
        n280 = Boolean Array To Number(Boolean array=w294) -> (number=w312:u32)
        n281 = Build Array (concatenate)("Channel \nHold Order", "Channel \nTransfer Order", w404, w399, w399, w399, w401, w400, w399, w399, w399, w276, "SoftDEMUX \nSelector Enable", "Channel DEMUX \nSelector", w277) -> (w286:bool[])
        n282 = Build Array (concatenate)(w482, bool[] [FALSE, FALSE, FALSE, FALSE] ("appended array"), w480, w480, "Time Reset") -> (w284:bool[])
        n283 = Boolean Array To Number(Boolean array=w290) -> (number=w308:u32)
        n284 = Boolean Array To Number(Boolean array=w315) -> (number=w318:u32)
        n285 = Boolean Array To Number(Boolean array=w288) -> (number=w306:u32)
        n286 = Number To Hexadecimal String(1:i16 8 ("width (-)"), 2:w310) -> (0:w291:string)
        "word2" <- w291
        n287 = Boolean Array To Number(Boolean array=w264) -> (number=w267:u32)
        n288 = Number To Hexadecimal String(1:i16 8 ("width (-)"), 2:w314) -> (0:w295:string)
        "word0" <- w295
        n289 = Number To Hexadecimal String(1:i16 8 ("width (-)"), 2:w312) -> (0:w293:string)
        "word1" <- w293
        n290 = Boolean Array To Number(Boolean array=w282) -> (number=w300:u32)
        n291 = Number To Hexadecimal String(1:i16 8 ("width (-)"), 2:w308) -> (0:w289:string)
        "word4" <- w289
        n292 = Boolean Array To Number(Boolean array=w284) -> (number=w302:u32)
        n293 = case shown="True" "Reset Register Map to Defaults" {
          tunnel: w270 -> [_ w618]
          tunnel: w272 -> [_ w617]
          tunnel: w278 -> [_ w616]
          frame False {
          }
          frame True {
            n294 = stacked-sequence {
              tunnel: w618 -> [w624 w632 w640 w648 w656 w664 w672 w680 w688 w696 w701]
              tunnel: w617 -> [w623 w631 w639 w647 w655 w663 w671 w679 w687 w695 w700]
              tunnel: w616 -> [w622 w630 w638 w646 w654 w662 w670 w678 w686 w694 _]
              frame #0 {
                n295 = call "RegisterMap2HexString.vi"("Word Num"=0, "string"=w622) -> ("concatenated string"=w621:string)  [unwired: 9 in]
                n296 = case shown="No Error" w623 {
                  tunnel: w624 -> [w627 _]
                  tunnel: w623 -> [w626 _]
                  tunnel: w621 -> [w625 _]
                  frame No Error {
                    n297 = Enqueue Element(queue=w627, element=w625, error in (no error)=w626) -> ()  [unwired: 1 in, 3 out]
                  }
                  frame Error {
                  }
                }
              }
              frame #1 {
                n298 = call "RegisterMap2HexString.vi"("Word Num"=1, "string"=w630) -> ("concatenated string"=w629:string)  [unwired: 9 in]
                n299 = case shown="No Error" w631 {
                  tunnel: w632 -> [w635 _]
                  tunnel: w631 -> [w634 _]
                  tunnel: w629 -> [w633 _]
                  frame No Error {
                    n300 = Enqueue Element(queue=w635, element=w633, error in (no error)=w634) -> ()  [unwired: 1 in, 3 out]
                  }
                  frame Error {
                  }
                }
              }
              frame #2 {
                n301 = call "RegisterMap2HexString.vi"("Word Num"=2, "string"=w638) -> ("concatenated string"=w637:string)  [unwired: 9 in]
                n302 = case shown="No Error" w639 {
                  tunnel: w640 -> [w643 _]
                  tunnel: w639 -> [w642 _]
                  tunnel: w637 -> [w641 _]
                  frame No Error {
                    n303 = Enqueue Element(queue=w643, element=w641, error in (no error)=w642) -> ()  [unwired: 1 in, 3 out]
                  }
                  frame Error {
                  }
                }
              }
              frame #3 {
                n304 = call "RegisterMap2HexString.vi"("Word Num"=3, "string"=w646) -> ("concatenated string"=w645:string)  [unwired: 9 in]
                n305 = case shown="No Error" w647 {
                  tunnel: w648 -> [w651 _]
                  tunnel: w647 -> [w650 _]
                  tunnel: w645 -> [w649 _]
                  frame No Error {
                    n306 = Enqueue Element(queue=w651, element=w649, error in (no error)=w650) -> ()  [unwired: 1 in, 3 out]
                  }
                  frame Error {
                  }
                }
              }
              frame #4 {
                n307 = call "RegisterMap2HexString.vi"("Word Num"=4, "string"=w654) -> ("concatenated string"=w653:string)  [unwired: 9 in]
                n308 = case shown="No Error" w655 {
                  tunnel: w656 -> [w659 _]
                  tunnel: w655 -> [w658 _]
                  tunnel: w653 -> [w657 _]
                  frame No Error {
                    n309 = Enqueue Element(queue=w659, element=w657, error in (no error)=w658) -> ()  [unwired: 1 in, 3 out]
                  }
                  frame Error {
                  }
                }
              }
              frame #5 {
                n310 = call "RegisterMap2HexString.vi"("Word Num"=5, "string"=w662) -> ("concatenated string"=w661:string)  [unwired: 9 in]
                n311 = case shown="No Error" w663 {
                  tunnel: w664 -> [w667 _]
                  tunnel: w663 -> [w666 _]
                  tunnel: w661 -> [w665 _]
                  frame No Error {
                    n312 = Enqueue Element(queue=w667, element=w665, error in (no error)=w666) -> ()  [unwired: 1 in, 3 out]
                  }
                  frame Error {
                  }
                }
              }
              frame #6 {
                n313 = call "RegisterMap2HexString.vi"("Word Num"=6, "string"=w670) -> ("concatenated string"=w669:string)  [unwired: 9 in]
                n314 = case shown="No Error" w671 {
                  tunnel: w672 -> [w675 _]
                  tunnel: w671 -> [w674 _]
                  tunnel: w669 -> [w673 _]
                  frame No Error {
                    n315 = Enqueue Element(queue=w675, element=w673, error in (no error)=w674) -> ()  [unwired: 1 in, 3 out]
                  }
                  frame Error {
                  }
                }
              }
              frame #7 {
                n316 = call "RegisterMap2HexString.vi"("Word Num"=7, "string"=w678) -> ("concatenated string"=w677:string)  [unwired: 9 in]
                n317 = case shown="No Error" w679 {
                  tunnel: w680 -> [w683 _]
                  tunnel: w679 -> [w682 _]
                  tunnel: w677 -> [w681 _]
                  frame No Error {
                    n318 = Enqueue Element(queue=w683, element=w681, error in (no error)=w682) -> ()  [unwired: 1 in, 3 out]
                  }
                  frame Error {
                  }
                }
              }
              frame #8 {
                n319 = call "RegisterMap2HexString.vi"("Word Num"=8, "string"=w686) -> ("concatenated string"=w685:string)  [unwired: 9 in]
                n320 = case shown="No Error" w687 {
                  tunnel: w688 -> [w691 _]
                  tunnel: w687 -> [w690 _]
                  tunnel: w685 -> [w689 _]
                  frame No Error {
                    n321 = Enqueue Element(queue=w691, element=w689, error in (no error)=w690) -> ()  [unwired: 1 in, 3 out]
                  }
                  frame Error {
                  }
                }
              }
              frame #9 {
                n322 = call "RegisterMap2HexString.vi"("Word Num"=9, "string"=w694) -> ("concatenated string"=w693:string)  [unwired: 9 in]
                n323 = case shown="No Error" w695 {
                  tunnel: w696 -> [w699 _]
                  tunnel: w695 -> [w698 _]
                  tunnel: w693 -> [w697 _]
                  frame No Error {
                    n324 = Enqueue Element(queue=w699, element=w697, error in (no error)=w698) -> ()  [unwired: 1 in, 3 out]
                  }
                  frame Error {
                  }
                }
              }
              frame #10 {
                n325 = case shown="No Error" w700 {
                  tunnel: w701 -> [w705 _]
                  tunnel: w700 -> [w704 _]
                  tunnel: "r0000000000" ("F-format string") -> [w703 _]
                  frame No Error {
                    n326 = Enqueue Element(queue=w705, element=w703, error in (no error)=w704) -> ()  [unwired: 1 in, 3 out]
                  }
                  frame Error {
                  }
                }
              }
            }
            n327 = local write "Reset Register Map to Defaults"(FALSE ("Read Register")) -> ()
            n328 = local write "Read Register"(TRUE ("Read Register")) -> ()
          }
        }
        n329 = Number To Hexadecimal String(1:i16 8 ("width (-)"), 2:w318) -> (0:w316:string)
        "word3" <- w316
        n330 = Number To Hexadecimal String(1:i16 8 ("width (-)"), 2:w306) -> (0:w287:string)
        "word5" <- w287
        n331 = Boolean Array To Number(Boolean array=w286) -> (number=w304:u32)
        n332 = Number To Hexadecimal String(1:i16 8 ("width (-)"), 2:w267) -> (0:w265:string)
        "word9" <- w265
        n333 = Number To Hexadecimal String(1:i16 8 ("width (-)"), 2:w300) -> (0:w281:string)
        "word8" <- w281
        n334 = Number To Hexadecimal String(1:i16 8 ("width (-)"), 2:w302) -> (0:w283:string)
        "word7" <- w283
        n335 = Number To Hexadecimal String(1:i16 8 ("width (-)"), 2:w304) -> (0:w285:string)
        "word6" <- w285
        n336 = Concatenate Strings("w09" ("string"), w265) -> (w268:string)
        n337 = Concatenate Strings("w00" ("string"), w295) -> (w448:string)
        n338 = Concatenate Strings("w02" ("string"), w291) -> (w435:string)
        n339 = Concatenate Strings("w01" ("string"), w293) -> (w436:string)
        n340 = Concatenate Strings("w03" ("string"), w316) -> (w319:string)
        n341 = Concatenate Strings("w05" ("string"), w287) -> (w433:string)
        n342 = Concatenate Strings("w04" ("string"), w289) -> (w434:string)
        n343 = Concatenate Strings("w06" ("string"), w285) -> (w432:string)
        n344 = Concatenate Strings("w0A" ("string"), w279) -> (w271:string)
        n345 = Concatenate Strings("w07" ("string"), w283) -> (w425:string)
        n346 = Concatenate Strings("w08" ("string"), w281) -> (w423:string)
        n347 = case shown="True" "Send Word 1" {
          tunnel: w436 -> [_ w588]
          tunnel: w270 -> [_ w586]
          tunnel: w272 -> [_ w587]
          frame False {
          }
          frame True {
            n348 = flat-sequence {
              tunnel: w587 -> [w592]
              tunnel: w586 -> [w591]
              tunnel: w588 -> [w590]
              tunnel: w586 -> [w598]
              tunnel: w587 -> [w597]
              tunnel: w587 -> [w603]
              tunnel: w586 -> [w602]
              frame #0 {
                n349 = case shown="No Error" w592 {
                  tunnel: w590 -> [w595 _]
                  tunnel: w592 -> [w594 _]
                  tunnel: w591 -> [w593 _]
                  frame No Error {
                    n350 = Enqueue Element(queue=w593, element=w595, error in (no error)=w594) -> ()  [unwired: 1 in, 3 out]
                  }
                  frame Error {
                  }
                }
              }
              frame #1 {
                n351 = case shown="No Error" w597 {
                  tunnel: w597 -> [w601 _]
                  tunnel: w598 -> [w600 _]
                  tunnel: "w0100000000" ("string") -> [w599 _]
                  frame No Error {
                    n352 = Enqueue Element(queue=w600, element=w599, error in (no error)=w601) -> ()  [unwired: 1 in, 3 out]
                  }
                  frame Error {
                  }
                }
              }
              frame #2 {
                n353 = case shown="No Error" w603 {
                  tunnel: w603 -> [w607 _]
                  tunnel: w602 -> [w606 _]
                  tunnel: "r0000000000" ("string") -> [w605 _]
                  frame No Error {
                    n354 = Enqueue Element(queue=w606, element=w605, error in (no error)=w607) -> ()  [unwired: 1 in, 3 out]
                  }
                  frame Error {
                  }
                }
              }
            }
            n355 = local write "Send Word 1"(FALSE ("Send")) -> ()
            n356 = local write "Read Register"(TRUE ("Read Register")) -> ()
          }
        }
        n357 = case shown="True" "Send Word 0" {
          tunnel: w448 -> [_ w611]
          tunnel: w270 -> [_ w610]
          tunnel: w272 -> [_ w608]
          frame False {
          }
          frame True {
            n358 = case shown="No Error" w608 {
              tunnel: w611 -> [w614 _]
              tunnel: w608 -> [w613 _]
              tunnel: w610 -> [w612 _]
              frame No Error {
                n359 = Enqueue Element(queue=w612, element=w614, error in (no error)=w613) -> ()  [unwired: 1 in, 3 out]
              }
              frame Error {
              }
            }
            n360 = local write "Send Word 0"(FALSE ("Send")) -> ()
          }
        }
        n361 = case shown="True" "Send Word 2" {
          tunnel: w435 -> [_ w581]
          tunnel: w270 -> [_ w580]
          tunnel: w272 -> [_ w578]
          frame False {
          }
          frame True {
            n362 = case shown="No Error" w578 {
              tunnel: w581 -> [w584 _]
              tunnel: w578 -> [w583 _]
              tunnel: w580 -> [w582 _]
              frame No Error {
                n363 = Enqueue Element(queue=w582, element=w584, error in (no error)=w583) -> ()  [unwired: 1 in, 3 out]
              }
              frame Error {
              }
            }
            n364 = local write "Send Word 2"(FALSE ("Send")) -> ()
          }
        }
        n365 = case shown="True" "Send Word 3" {
          tunnel: w319 -> [_ w574]
          tunnel: w270 -> [_ w573]
          tunnel: w272 -> [_ w571]
          frame False {
          }
          frame True {
            n366 = case shown="No Error" w571 {
              tunnel: w574 -> [w577 _]
              tunnel: w571 -> [w576 _]
              tunnel: w573 -> [w575 _]
              frame No Error {
                n367 = Enqueue Element(queue=w575, element=w577, error in (no error)=w576) -> ()  [unwired: 1 in, 3 out]
              }
              frame Error {
              }
            }
            n368 = local write "Send Word 3"(FALSE ("Send")) -> ()
          }
        }
        n369 = case shown="True" "Send Word 4" {
          tunnel: w434 -> [_ w567]
          tunnel: w270 -> [_ w566]
          tunnel: w272 -> [_ w564]
          frame False {
          }
          frame True {
            n370 = case shown="No Error" w564 {
              tunnel: w567 -> [w570 _]
              tunnel: w564 -> [w569 _]
              tunnel: w566 -> [w568 _]
              frame No Error {
                n371 = Enqueue Element(queue=w568, element=w570, error in (no error)=w569) -> ()  [unwired: 1 in, 3 out]
              }
              frame Error {
              }
            }
            n372 = local write "Send Word 4"(FALSE ("Send")) -> ()
          }
        }
        n373 = case shown="True" "Send Word 5" {
          tunnel: w433 -> [_ w560]
          tunnel: w270 -> [_ w559]
          tunnel: w272 -> [_ w557]
          frame False {
          }
          frame True {
            n374 = case shown="No Error" w557 {
              tunnel: w560 -> [w563 _]
              tunnel: w557 -> [w562 _]
              tunnel: w559 -> [w561 _]
              frame No Error {
                n375 = Enqueue Element(queue=w561, element=w563, error in (no error)=w562) -> ()  [unwired: 1 in, 3 out]
              }
              frame Error {
              }
            }
            n376 = local write "Send Word 5"(FALSE ("Send")) -> ()
          }
        }
        n377 = case shown="True" "Send Word 6" {
          tunnel: w432 -> [_ w553]
          tunnel: w270 -> [_ w552]
          tunnel: w272 -> [_ w550]
          frame False {
          }
          frame True {
            n378 = case shown="No Error" w550 {
              tunnel: w553 -> [w556 _]
              tunnel: w550 -> [w555 _]
              tunnel: w552 -> [w554 _]
              frame No Error {
                n379 = Enqueue Element(queue=w554, element=w556, error in (no error)=w555) -> ()  [unwired: 1 in, 3 out]
              }
              frame Error {
              }
            }
            n380 = local write "Send Word 6"(FALSE ("Send")) -> ()
          }
        }
        n381 = case shown="True" "Send Word 7" {
          tunnel: w425 -> [_ w546]
          tunnel: w270 -> [_ w545]
          tunnel: w272 -> [_ w543]
          frame False {
          }
          frame True {
            n382 = case shown="No Error" w543 {
              tunnel: w546 -> [w549 _]
              tunnel: w543 -> [w548 _]
              tunnel: w545 -> [w547 _]
              frame No Error {
                n383 = Enqueue Element(queue=w547, element=w549, error in (no error)=w548) -> ()  [unwired: 1 in, 3 out]
              }
              frame Error {
              }
            }
            n384 = local write "Send Word 7"(FALSE ("Send")) -> ()
          }
        }
        n385 = case shown="True" "Send Word 8" {
          tunnel: w423 -> [_ w539]
          tunnel: w270 -> [_ w538]
          tunnel: w272 -> [_ w536]
          frame False {
          }
          frame True {
            n386 = case shown="No Error" w536 {
              tunnel: w539 -> [w542 _]
              tunnel: w536 -> [w541 _]
              tunnel: w538 -> [w540 _]
              frame No Error {
                n387 = Enqueue Element(queue=w540, element=w542, error in (no error)=w541) -> ()  [unwired: 1 in, 3 out]
              }
              frame Error {
              }
            }
            n388 = local write "Send Word 8"(FALSE ("Send")) -> ()
          }
        }
        n389 = case shown="True" "Send Word 9" {
          tunnel: w268 -> [_ w532]
          tunnel: w270 -> [_ w531]
          tunnel: w272 -> [_ w529]
          frame False {
          }
          frame True {
            n390 = case shown="No Error" w529 {
              tunnel: w532 -> [w535 _]
              tunnel: w529 -> [w534 _]
              tunnel: w531 -> [w533 _]
              frame No Error {
                n391 = Enqueue Element(queue=w533, element=w535, error in (no error)=w534) -> ()  [unwired: 1 in, 3 out]
              }
              frame Error {
              }
            }
            n392 = local write "Send Word 9"(FALSE ("Send")) -> ()
          }
        }
        n393 = case shown="True" "Send Word A" {
          tunnel: w271 -> [_ w525]
          tunnel: w270 -> [_ w524]
          tunnel: w272 -> [_ w522]
          frame False {
          }
          frame True {
            n394 = case shown="No Error" w522 {
              tunnel: w525 -> [w528 _]
              tunnel: w522 -> [w527 _]
              tunnel: w524 -> [w526 _]
              frame No Error {
                n395 = Enqueue Element(queue=w526, element=w528, error in (no error)=w527) -> ()  [unwired: 1 in, 3 out]
              }
              frame Error {
              }
            }
            n396 = local write "Send Word A"(FALSE ("Send")) -> ()
          }
        }
      }
    }
  }
